vi "Code stuff and things.vi"(11 "Lines (Shape Detection 1) in":T1(array[cluster])) -> (0 "Predicted Y Coordinates":sgl, 1 "Predicted X Coordinates":sgl, 2 "Dun Fuk Up?":bool, 3 "Chosen Y":sgl)   [LabVIEW 2012]
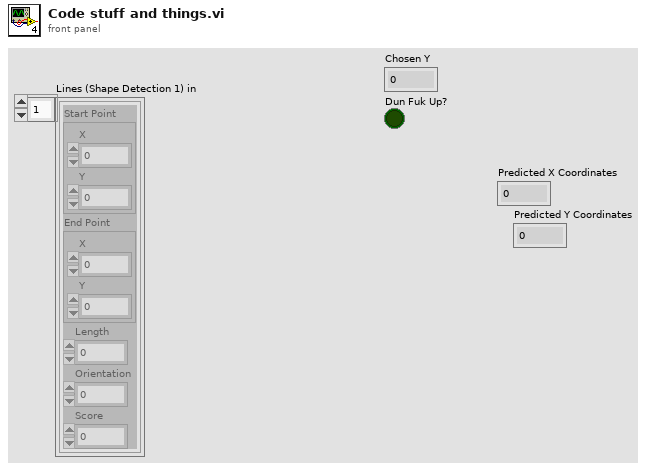
[diagram p1: front panel]
types:
  T1 = cluster{"Start Point":cluster{"X":sgl, "Y":sgl}, "End Point":cluster{"X":sgl, "Y":sgl}, "Length":dbl, "Orientation":dbl, "Score":dbl}[]
  T2 = cluster{"Lines (Shape Detection 1) in[0]":cluster{"Start Point":cluster{"X":sgl, "Y":sgl}, "End Point":cluster{"X":sgl, "Y":sgl}, "Length":dbl, "Orientation":dbl, "Score":dbl}, "Lines (Shape Detection 1) in[1]":cluster{"Start Point":cluster{"X":sgl, "Y":sgl}, "End Point":cluster{"X":sgl, "Y":sgl}, "Length":dbl, "Orientation":dbl, "Score":dbl}, "Lines (Shape Detection 1) in[2]":cluster{"Start Point":cluster{"X":sgl, "Y":sgl}, "End Point":cluster{"X":sgl, "Y":sgl}, "Length":dbl, "Orientation":dbl, "Score":dbl}, "Lines (Shape Detection 1) in[3]":cluster{"Start Point":cluster{"X":sgl, "Y":sgl}, "End Point":cluster{"X":sgl, "Y":sgl}, "Length":dbl, "Orientation":dbl, "Score":dbl}, "Lines (Shape Detection 1) in[4]":cluster{"Start Point":cluster{"X":sgl, "Y":sgl}, "End Point":cluster{"X":sgl, "Y":sgl}, "Length":dbl, "Orientation":dbl, "Score":dbl}, "Lines (Shape Detection 1) in[5]":cluster{"Start Point":cluster{"X":sgl, "Y":sgl}, "End Point":cluster{"X":sgl, "Y":sgl}, "Length":dbl, "Orientation":dbl, "Score":dbl}, "Lines (Shape Detection 1) in[6]":cluster{"Start Point":cluster{"X":sgl, "Y":sgl}, "End Point":cluster{"X":sgl, "Y":sgl}, "Length":dbl, "Orientation":dbl, "Score":dbl}, "Lines (Shape Detection 1) in[7]":cluster{"Start Point":cluster{"X":sgl, "Y":sgl}, "End Point":cluster{"X":sgl, "Y":sgl}, "Length":dbl, "Orientation":dbl, "Score":dbl}, "Lines (Shape Detection 1) in[8]":cluster{"Start Point":cluster{"X":sgl, "Y":sgl}, "End Point":cluster{"X":sgl, "Y":sgl}, "Length":dbl, "Orientation":dbl, "Score":dbl}}
  T3 = cluster{"Start Point":cluster{"X":sgl, "Y":sgl}, "End Point":cluster{"X":sgl, "Y":sgl}, "Length":dbl, "Orientation":dbl, "Score":dbl}
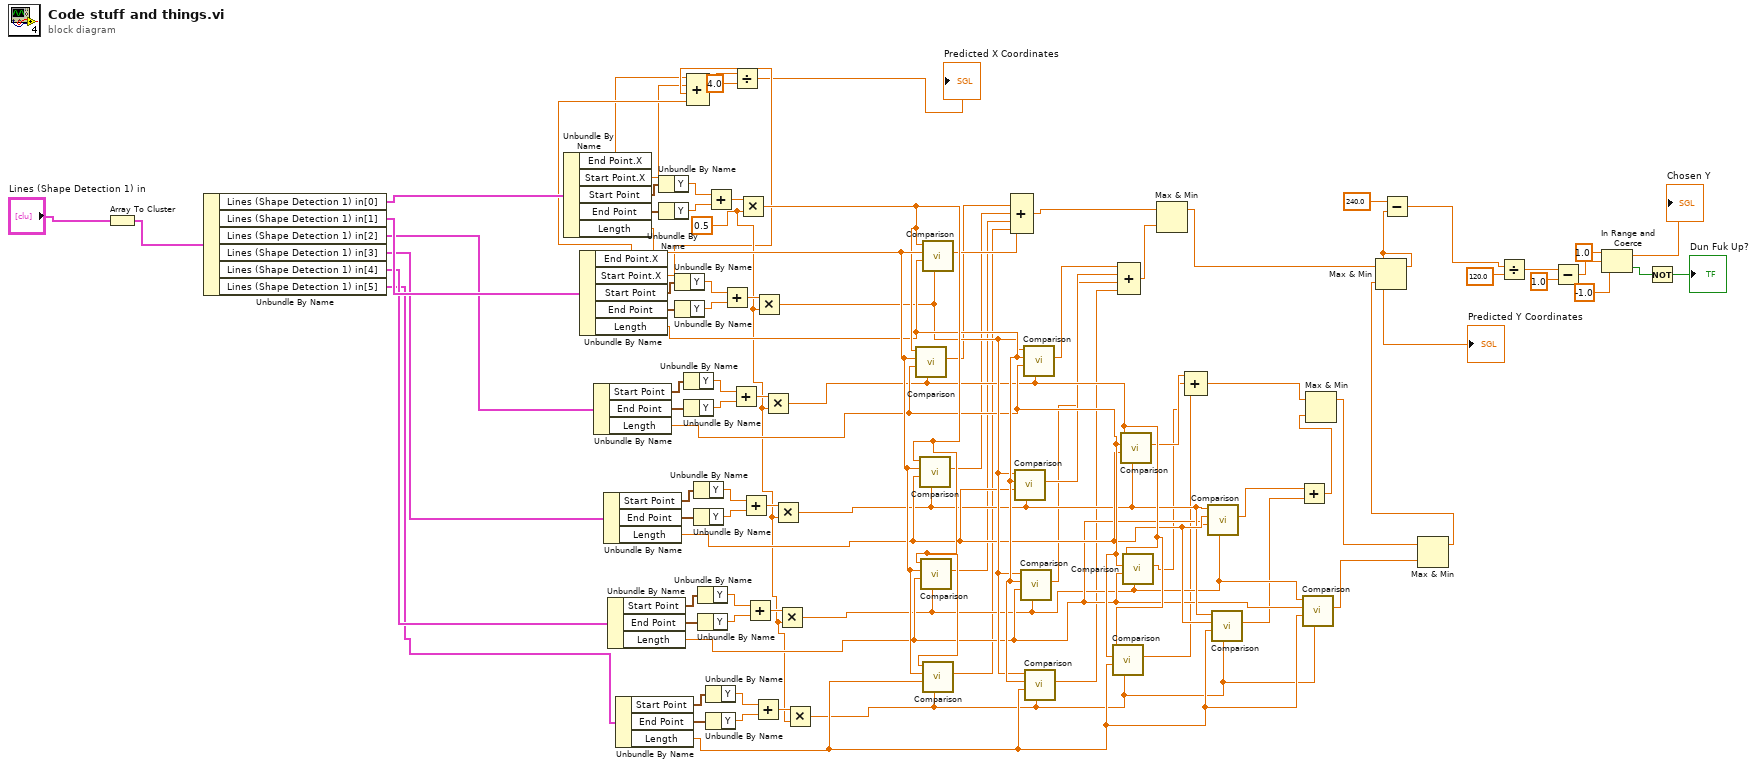
[diagram p0: block diagram]
diagram:
  w23 = sgl 0.5 ("y")
  n1 = Array To Cluster(array="Lines (Shape Detection 1) in") -> (cluster=w91:T2)
  n2 = Unbundle By Name(w91) -> ("Lines (Shape Detection 1) in[0]"=w90:T3, "Lines (Shape Detection 1) in[1]"=w59:T3, "Lines (Shape Detection 1) in[2]"=w58:T3, "Lines (Shape Detection 1) in[3]"=w57:T3, "Lines (Shape Detection 1) in[4]"=w56:T3, "Lines (Shape Detection 1) in[5]"=w55:T3)
  n3 = Unbundle By Name(w90) -> ("End Point.X"=w4:sgl, "Start Point.X"=w5:sgl, "Start Point"=w89:cluster{"X":sgl, "Y":sgl}, "End Point"=w88:cluster{"X":sgl, "Y":sgl}, "Length"=w54:dbl)
  n4 = Unbundle By Name(w59) -> ("End Point.X"=w7:sgl, "Start Point.X"=w6:sgl, "Start Point"=w84:cluster{"X":sgl, "Y":sgl}, "End Point"=w83:cluster{"X":sgl, "Y":sgl}, "Length"=w52:dbl)
  n5 = Unbundle By Name(w58) -> ("Start Point"=w79:cluster{"X":sgl, "Y":sgl}, "End Point"=w78:cluster{"X":sgl, "Y":sgl}, "Length"=w50:dbl)
  n6 = Unbundle By Name(w57) -> ("Start Point"=w74:cluster{"X":sgl, "Y":sgl}, "End Point"=w73:cluster{"X":sgl, "Y":sgl}, "Length"=w48:dbl)
  n7 = Unbundle By Name(w56) -> ("Start Point"=w69:cluster{"X":sgl, "Y":sgl}, "End Point"=w68:cluster{"X":sgl, "Y":sgl}, "Length"=w46:dbl)
  n8 = Unbundle By Name(w55) -> ("Start Point"=w64:cluster{"X":sgl, "Y":sgl}, "End Point"=w63:cluster{"X":sgl, "Y":sgl}, "Length"=w45:dbl)
  n9 = Unbundle By Name(w89) -> ("Y"=w86:sgl)
  n10 = Unbundle By Name(w88) -> ("Y"=w87:sgl)
  n11 = Unbundle By Name(w84) -> ("Y"=w81:sgl)
  n12 = Unbundle By Name(w83) -> ("Y"=w82:sgl)
  n13 = Unbundle By Name(w79) -> ("Y"=w76:sgl)
  n14 = Unbundle By Name(w78) -> ("Y"=w77:sgl)
  n15 = Compound Arithmetic op=ADD(w4, w5, w6, w7) -> (w3:sgl)
  n16 = Unbundle By Name(w74) -> ("Y"=w71:sgl)
  n17 = Unbundle By Name(w73) -> ("Y"=w72:sgl)
  n18 = Unbundle By Name(w69) -> ("Y"=w66:sgl)
  n19 = Unbundle By Name(w68) -> ("Y"=w67:sgl)
  n20 = Add(x=w86, y=w87) -> (x+y=w85:sgl)
  n21 = Unbundle By Name(w64) -> ("Y"=w61:sgl)
  n22 = Unbundle By Name(w63) -> ("Y"=w62:sgl)
  n23 = Add(x=w81, y=w82) -> (x+y=w80:sgl)
  n24 = Add(x=w76, y=w77) -> (x+y=w75:sgl)
  n25 = Divide(x=w3, y=sgl 4.0) -> (x/y=→"Predicted X Coordinates":sgl)
  n26 = Multiply(x=w85, y=w23) -> (x*y=w53:sgl)
  n27 = Add(x=w71, y=w72) -> (x+y=w70:sgl)
  n28 = Add(x=w66, y=w67) -> (x+y=w65:sgl)
  n29 = Add(x=w61, y=w62) -> (x+y=w60:sgl)
  n30 = Multiply(x=w80, y=w23) -> (x*y=w51:sgl)
  n31 = Multiply(x=w75, y=w23) -> (x*y=w49:sgl)
  n32 = Multiply(x=w70, y=w23) -> (x*y=w47:sgl)
  n33 = Multiply(x=w65, y=w23) -> (x*y=w44:sgl)
  n34 = Multiply(x=w60, y=w23) -> (x*y=w43:sgl)
  n35 = call "Comparison.vi"("Y2"=w49, "Length 2"=w50, "Length"=w54, "Y1"=w53) -> ("Output"=w41:sgl)  [unwired: 7 in]
  n36 = call "Comparison.vi"("Y2"=w47, "Length 2"=w48, "Length"=w54, "Y1"=w53) -> ("Output"=w40:sgl)  [unwired: 7 in]
  n37 = call "Comparison.vi"("Y2"=w44, "Length 2"=w46, "Length"=w54, "Y1"=w53) -> ("Output"=w39:sgl)  [unwired: 7 in]
  n38 = call "Comparison.vi"("Y2"=w51, "Length 2"=w52, "Length"=w54, "Y1"=w53) -> ("Output"=w42:sgl)  [unwired: 7 in]
  n39 = call "Comparison.vi"("Y2"=w43, "Length 2"=w45, "Length"=w54, "Y1"=w53) -> ("Output"=w38:sgl)  [unwired: 7 in]
  n40 = Compound Arithmetic op=ADD(w42, w41, w40, w39, w38) -> (w28:sgl)
  n41 = call "Comparison.vi"("Y2"=w47, "Length 2"=w48, "Length"=w52, "Y1"=w51) -> ("Output"=w36:sgl)  [unwired: 7 in]
  n42 = call "Comparison.vi"("Y2"=w44, "Length 2"=w46, "Length"=w52, "Y1"=w51) -> ("Output"=w35:sgl)  [unwired: 7 in]
  n43 = call "Comparison.vi"("Y2"=w49, "Length 2"=w50, "Length"=w52, "Y1"=w51) -> ("Output"=w37:sgl)  [unwired: 7 in]
  n44 = call "Comparison.vi"("Y2"=w43, "Length 2"=w45, "Length"=w52, "Y1"=w51) -> ("Output"=w34:sgl)  [unwired: 7 in]
  n45 = call "Comparison.vi"("Y2"=w43, "Length 2"=w45, "Length"=w50, "Y1"=w49) -> ("Output"=w31:sgl)  [unwired: 7 in]
  n46 = Compound Arithmetic op=ADD(w37, w36, w35, w34) -> (w27:sgl)
  n47 = call "Comparison.vi"("Y2"=w47, "Length 2"=w48, "Length"=w50, "Y1"=w49) -> ("Output"=w33:sgl)  [unwired: 7 in]
  n48 = call "Comparison.vi"("Y2"=w44, "Length 2"=w46, "Length"=w50, "Y1"=w49) -> ("Output"=w32:sgl)  [unwired: 7 in]
  n49 = Max & Min(x=w28, y=w27) -> (max(x,y)=w17:sgl)  [unwired: 1 out]
  n50 = Compound Arithmetic op=ADD(w33, w32, w31) -> (w26:sgl)
  n51 = call "Comparison.vi"("Y2"=w44, "Length 2"=w46, "Length"=w48, "Y1"=w47) -> ("Output"=w30:sgl)  [unwired: 7 in]
  n52 = call "Comparison.vi"("Y2"=w43, "Length 2"=w45, "Length"=w48, "Y1"=w47) -> ("Output"=w29:sgl)  [unwired: 7 in]
  n53 = Add(x=w30, y=w29) -> (x+y=w25:sgl)
  n54 = call "Comparison.vi"("Y2"=w43, "Length 2"=w45, "Length"=w46, "Y1"=w44) -> ("Output"=w24:sgl)  [unwired: 7 in]
  n55 = Max & Min(x=w26, y=w25) -> (max(x,y)=w16:sgl)  [unwired: 1 out]
  n56 = Max & Min(x=w16, y=w24) -> (max(x,y)=w15:sgl)  [unwired: 1 out]
  n57 = Max & Min(x=w17, y=w15) -> (max(x,y)=w14:sgl)  [unwired: 1 out]
  "Predicted Y Coordinates" <- w14
  n58 = Subtract(x=240.0, y=w14) -> (x-y=w18:dbl)
  n59 = Divide(x=w18, y=sgl 120.0) -> (x/y=w21:dbl)
  n60 = Subtract(x=w21, y=sgl 1.0) -> (x-y=w13:dbl)
  n61 = In Range and Coerce(upper limit=1.0, x=w13, lower limit=-1.0) -> (coerced(x)=→"Chosen Y":dbl, In Range?=w9:bool)
  n62 = Not(x=w9) -> (.not. x?=→"Dun Fuk Up?":bool)
